vi "4-k-invdist.vi"(8 "err in":errorcluster, 9 "F(k)":dbl, 11 "p_Pois.":T1 caption="p_POI") -> (0 "err out":errorcluster caption="err  out", 1 "F(k)":dbl, 2 "k":dbl, 3 "p_Bin (s)":T1, 5 "k interpolé":dbl)   [LabVIEW 2010, in "lv_02.lvlib"]
uses:
  p_5E4_LBin.ctl
  <vilib>/gmath/statdist.llb/Binomial Inverse CDF.vi
  lv_02.lvlib
  <vilib>/gmath/NI_Gmath.lvlib
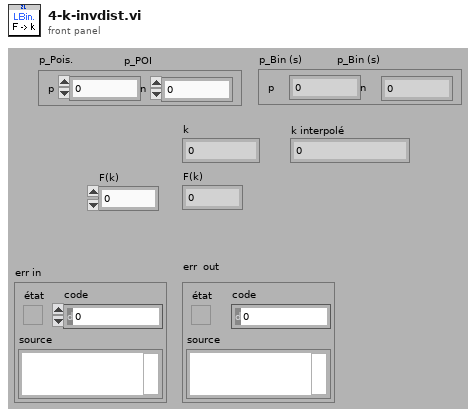
[diagram p1: front panel]
types:
  T1 = typedef "lv_02.lvlib/p_5E4_LBin.ctl" = cluster{"p":dbl, "n":i16}
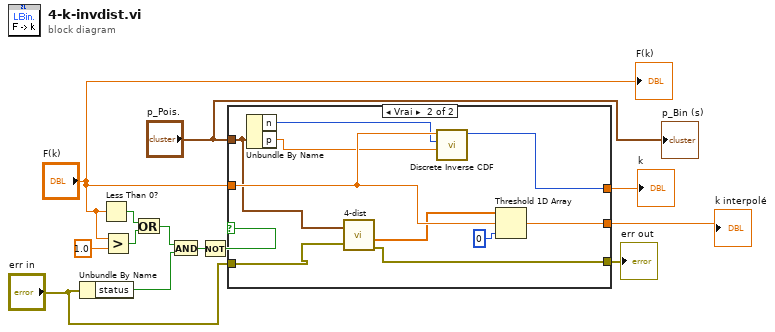
[diagram p0: block diagram]
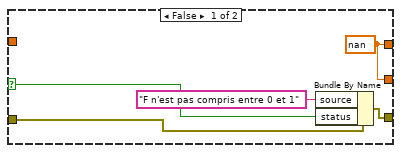
[diagram p2: hidden frame]
diagram:
  n1 = Unbundle By Name("err in") -> ("status"=w7:bool)
  n2 = Less Than 0?(x="F(k)") -> (x < 0?=w9:bool)
  n3 = Greater?(x="F(k)", y=1.0) -> (0:w10:bool)
  n4 = Or(x=w9, y=w10) -> (x .or. y?=w8:bool)
  n5 = And(x=w8, y=w7) -> (x .and. y?=w6:bool)
  n6 = Not(x=w6) -> (.not. x?=w5:bool)
  n7 = case shown="Vrai" w5 {
    selector: w5 -> [w16 _]
    tunnel: "F(k)" -> [_ w25]
    tunnel: [w14 w28] -> w13
    tunnel: "err in" -> [w17 w23]
    tunnel: [w18 w22] -> w3
    tunnel: "p_Pois." -> [_ w24]
    tunnel: [w14 w26] -> w1
    frame False {
      w14 = nan ("x")
      n8 = Bundle By Name(cluster=w17, "source"="F n'est pas compris entre 0 et 1", "status"=w16) -> (w18:errorcluster)
    }
    frame True {
      n9 = Unbundle By Name(w24) -> ("n"=w19:i16, "p"=w20:dbl)
      n10 = call "4-dist.vi"("err in 2"=w23, "p_LBin"=w24) -> ("err in"=w22:errorcluster, "F"=w21:dbl[])  [unwired: 2 out]
      n11 = call-poly <vilib>:"Discrete Inverse CDF.vi"("p"=w20, "n"=w19, "cdf(x)"=w25) -> ("x"=w28:i32)  [unwired: 7 in, 1 out]
      n12 = Threshold 1D Array(1:0 ("indice de départ (0)"), 2:w25, 3:w21) -> (0:w26:dbl)
    }
  }
  "k" <- w13
  "err out" <- w3
  "k interpolé" <- w1
  "F(k)" <- "F(k)"
  "p_Bin (s)" <- "p_Pois."
